vi "Graphical Test Runner - App Data Subvi.vi"() -> (0 "SMUI Template App Data":T1)   [LabVIEW 2009, in "GraphicalTestRunner.lvlib"]
uses:
  GraphicalTestRunner.lvlib
  Graphical Test Runner - App Data.ctl
  Classes/TextTestRunner/TextTestRunner.lvclass
  Classes/TestSuite/TestSuite.lvclass
  Classes/TestResult/resultStatusChanged--Cluster.ctl
  Classes/TestResult/resultStatus--enum.ctl
  Classes/TestSuite/suiteStatusChanged--Cluster.ctl
  Classes/TestSuite/suiteStatus--enum.ctl
  Classes/TestCase/TestCase.lvclass
  <userlib>/_OpenG.lib/dictionary/dictionary.llb/Dictionary Object RefNum__ogtk.ctl
  <userlib>/_OpenG.lib/dictionary/dictionary.llb/Dictionary Object RefNum - Enum__ogtk.ctl
  Classes/TestResult/TestResult.lvclass
panel:
  # "Copyright © 2007 James Kring, Inc. All rights reserved.\n\nAuthor: Omar Mussa [omar.mussa@jameskring.com]\n\nThis library is provided \"AS IS\" ,WITHOUT WARRANTIES OR \nCONDITIONS OF ANY KIND, either express or implied.\n\nJames Kring, Inc. -- http://www.jameskring.com"
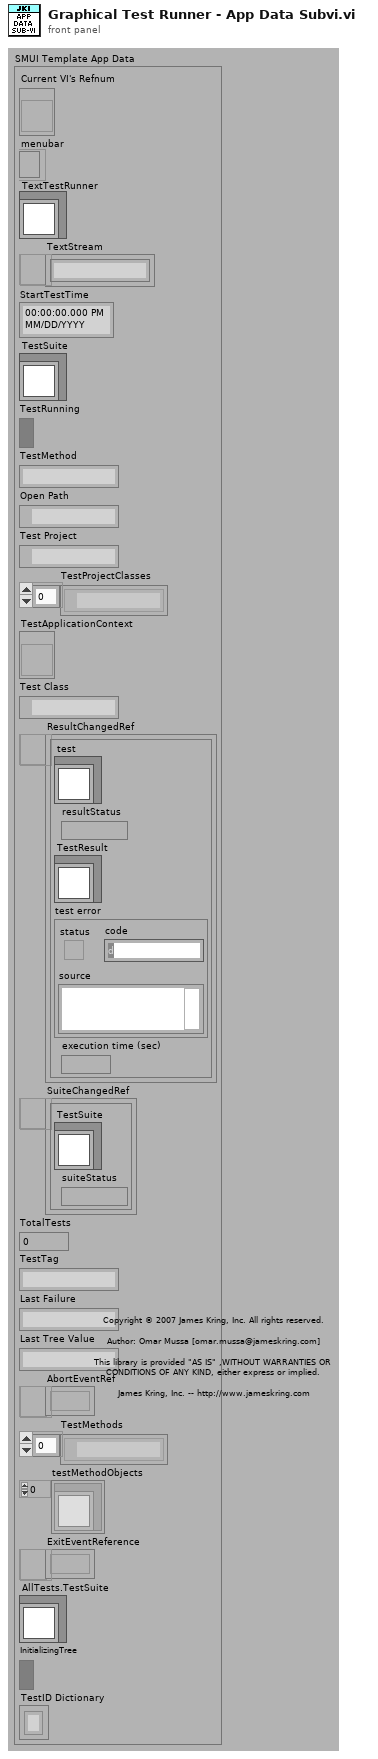
[diagram p1: front panel]
types:
  T1 = typedef "GraphicalTestRunner.lvlib/Graphical Test Runner - App Data.ctl" = cluster{"Current VI's Refnum":refnum<vi>, "menubar":refnum<k9>, "TextTestRunner":refnum<class "TextTestRunner.lvclass">, "TextStream":refnum<queue>, "StartTestTime":timestamp, "TestSuite":refnum<class "TestSuite.lvclass">, "TestRunning":bool, "TestMethod":string, "Open Path":path, "Test Project":path, "TestProjectClasses":path[], "TestApplicationContext":refnum<vi>, "Test Class":path, "ResultChangedRef":refnum<user-event>, "SuiteChangedRef":refnum<user-event>, "TotalTests":i32, "TestTag":string, "Last Failure":string, "Last Tree Value":string, "AbortEventRef":refnum<user-event>, "TestMethods":path[], "testMethodObjects":refnum<class "TestCase.lvclass">[], "ExitEventReference":refnum<user-event>, "AllTests.TestSuite":refnum<class "TestSuite.lvclass">, "InitializingTree":bool, "TestID Dictionary":T2}
  T2 = typedef "Dictionary Object RefNum__ogtk.ctl" = refnum<k1>
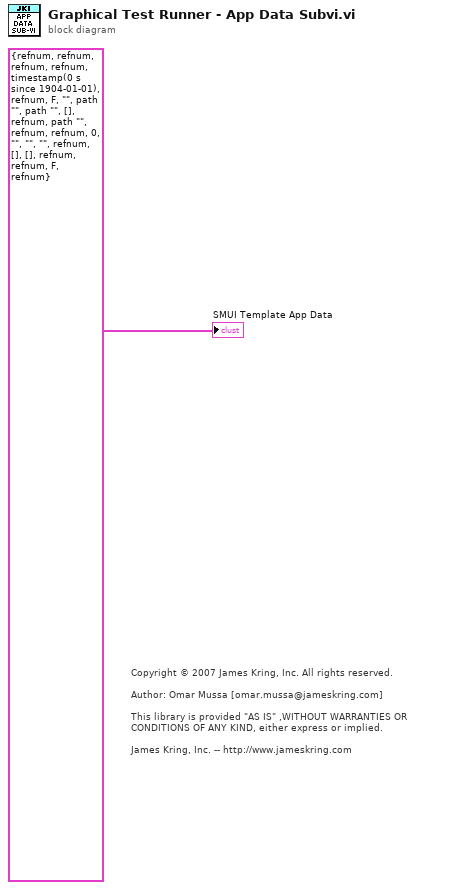
[diagram p0: block diagram]
diagram:
  # "Copyright © 2007 James Kring, Inc. All rights reserved.\n\nAuthor: Omar Mussa [omar.mussa@jameskring.com]\n\nThis library is provided \"AS IS\" ,WITHOUT WARRANTIES OR \nCONDITIONS OF ANY KIND, either express or implied.\n\nJames Kring, Inc. -- http://www.jameskring.com"
  "SMUI Template App Data" <- T1 {"Current VI's Refnum"=refnum, "menubar"=refnum, "TextTestRunner"=refnum, "TextStream"=refnum, "StartTestTime"=timestamp(0 s since 1904-01-01), "TestSuite"=refnum, "TestRunning"=FALSE, "TestMethod"="", "Open Path"=path "", "Test Project"=path "", "TestProjectClasses"=[], "TestApplicationContext"=refnum, "Test Class"=path "", "ResultChangedRef"=refnum, "SuiteChangedRef"=refnum, "TotalTests"=0, "TestTag"="", "Last Failure"="", "Last Tree Value"="", "AbortEventRef"=refnum, "TestMethods"=[], "testMethodObjects"=[], "ExitEventReference"=refnum, "AllTests.TestSuite"=refnum, "InitializingTree"=FALSE, "TestID Dictionary"=refnum} ("SMUI Template App Data")
